vi "Network_Cycle_Shared_Variables_v4.vi"(1 "error in (no error)":errorcluster, 2 "Igor Instruction String":string[](array[string])) -> (0 "error out":errorcluster)   [LabVIEW 2013, in "Labview_Networking.lvlib"]
doc: "Uses DataSocket technology to write live images."
uses:
  Labview_Networking.lvlib
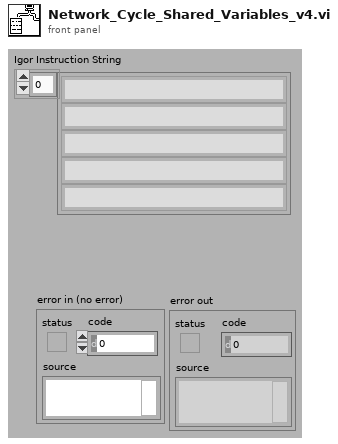
[diagram p1: front panel]
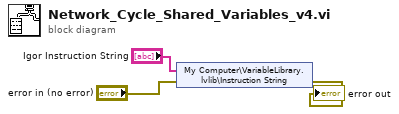
[diagram p0: block diagram]
diagram:
  n1 = shared-variable "My Computer\\VariableLibrary.lvlib\\Instruction String"("Igor Instruction String", error in="error in (no error)") -> (error out=→"error out":errorcluster)
